vi "seno.vi"() -> ()   [LabVIEW 2013]
panel:
  in  "frecuencia":dbl(knob) scale=0.0..100.0
  in  "amplitud":dbl(knob) scale=-10.0..10.0
  in  "Numero de Interacciones":dbl
  out "Waveform Graph":dbl[](graph)
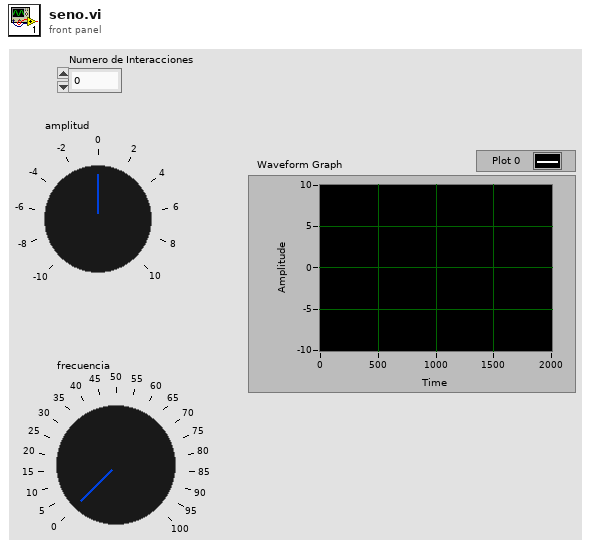
[diagram p1: front panel]
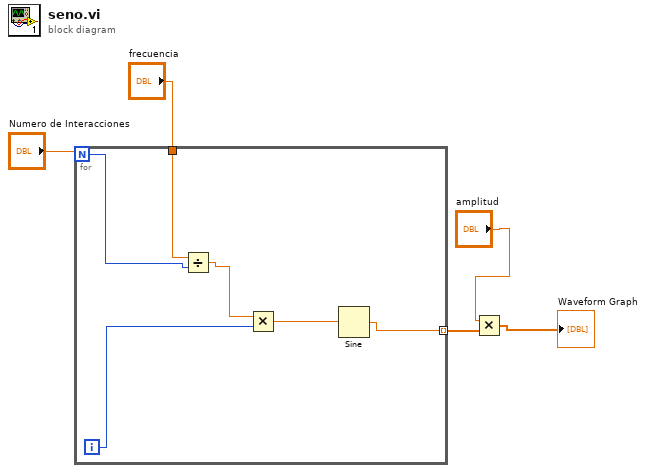
[diagram p0: block diagram]
diagram:
  n1 = for {
    N: "Numero de Interacciones" -> [w8]
    tunnel: [w7] -> w4 mode=indexing
    tunnel: "frecuencia" -> [w6]
    i -> [w10]
    n2 = Divide(x=w6, y=w8) -> (x/y=w9:dbl)
    n3 = Multiply(x=w9, y=w10) -> (x*y=w11:dbl)
    n4 = Sine(x=w11) -> (sin(x)=w7:dbl)
  }
  n5 = Multiply(x="amplitud", y=w4) -> (x*y=→"Waveform Graph":dbl[])
